vi "RSS addons filter.vi"(9 "add-ons":T1[](array[typedef]) {"component type" items=["standard", "hidden", "system", "unknown", "startup", "image"]}) -> (1 "add-ons out":T1[](array[typedef]) {"component type" items=["standard", "hidden", "system", "unknown", "startup", "image"]})   [LabVIEW 2015, in "RT Management.lvlib" / "RT Management.lvclass"]
uses:
  RT Management.lvclass
  <vilib>/nisyscfg/Software 1.2.ctl
  <vilib>/nisyscfg/Component Type.ctl
  <vilib>/nisyscfg/nisyscfg.lvlib
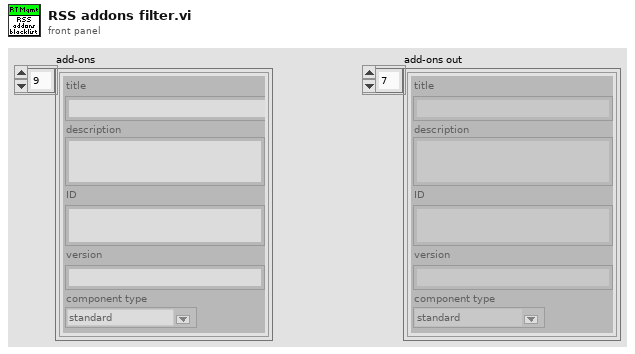
[diagram p1: front panel]
types:
  T1 = typedef "nisyscfg.lvlib/Software 1.2.ctl" = cluster{"title":string, "description":string, "ID":string, "version":string, "component type":T2}
  T2 = typedef "nisyscfg.lvlib/Component Type.ctl" = u32
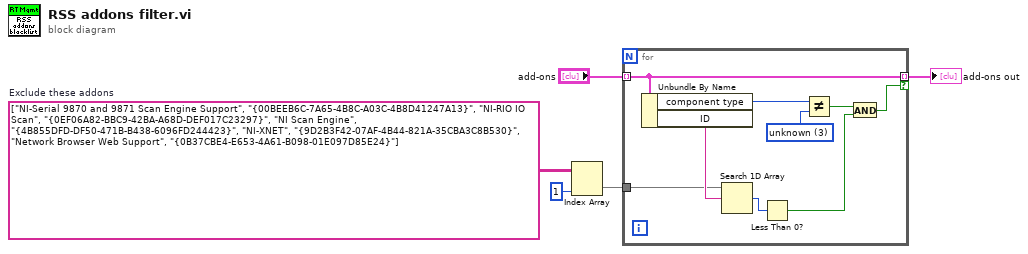
[diagram p0: block diagram]
diagram:
  w3 = string[][] [["NI-Serial 9870 and 9871 Scan Engine Support", "{00BEEB6C-7A65-4B8C-A03C-4B8D41247A13}"], ["NI-RIO IO Scan", "{0EF06A82-BBC9-42BA-A68D-DEF017C23297}"], ["NI Scan Engine", "{4B855DFD-DF50-471B-B438-6096FD244423}"], ["NI-XNET", "{9D2B3F42-07AF-4B44-821A-35CBA3C8B530}"], ["Network Browser Web Support", "{0B37CBE4-E653-4A61-B098-01E097D85E24}"]]  # Exclude these addons
  n1 = Index Array(array=w3, index (col)=1 ("disabled index (col)")) -> (element=w1:string[])  [unwired: 1 in]
  n2 = for {
    tunnel: "add-ons" -> [w12] mode=indexing
    tunnel: [w12] -> w4 mode=indexing if=w8
    tunnel: w1 -> [w6]
    w14 = T2 3 items=["standard", "hidden", "system", "unknown", "startup", "image"] ("component type")
    n3 = Unbundle By Name(w12) -> ("component type"=w13:T2, "ID"=w7:string)
    n4 = Search 1D Array(1D array=w6, element=w7) -> (index of element=w11:i32)  [unwired: 1 in]
    n5 = Less Than 0?(x=w11) -> (x < 0?=w9:bool)
    n6 = Not Equal?(x=w13, y=w14) -> (x != y?=w10:bool)
    n7 = And(x=w10, y=w9) -> (x .and. y?=w8:bool)
  }
  "add-ons out" <- w4
